vi "MenuEditor.vi"(11 "ItemsIn":T1(array[cluster])) -> (0 "Cancelled?":bool, 3 "ItemsOut":T1(array[cluster]))   [LabVIEW 2020, in "XMenuBar.xctl"]
doc: "Menu Item Editor"
uses:
  XMenuBar.xctl
panel:
  in  "Down":bool
  in  "Up":bool
  in  "Png":bool
  in  "LvSymb":i32(listbox)
  in  "PngSymb":path
  in  "IndentIn":bool
  in  "IndentOut":bool
  in  "Remove":bool
  in  "Add":bool
  in  "ItemTag":string caption="Item Tag:"
  in  "Checked":bool
  in  "ParentTag":string caption="Parent Tag(Use empty for top level menue):"
  in  "Load":bool
  in  "Name":string caption="ItemName"
  in  "Save":bool
  in  "Data":string(tree) caption="XMenu Data:"
  in  "Cancel":bool
  in  "OK":bool
  # "Item Operation"
  # "Menu File"
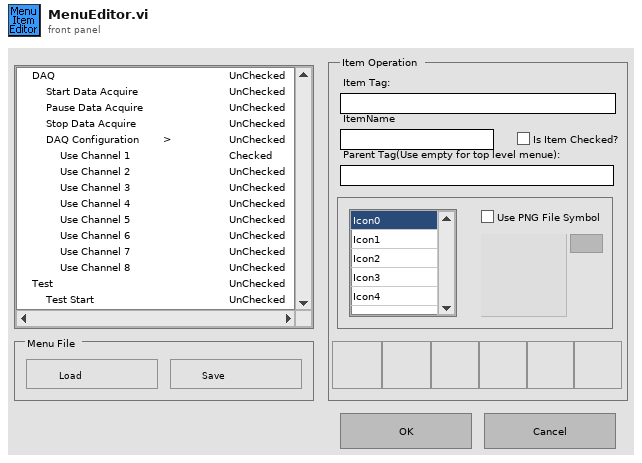
[diagram p1: front panel]
types:
  T1 = cluster{"Tag":string, "Name":string, "Index":i32, "Checked":bool, "Parent":string}[]
  T2 = enum16{"open", "replace", "create", "open or create", "replace or create", "replace or create with confirmation"}
  T3 = cluster{"Tag":string, "Name":string, "Symbol":i32, "Checked":bool, "ParentTag":string}
  T4 = enum8{"Enabled", "Disabled", "Disabled and Grayed Out"}
  T5 = typedef "imagedata.ctl" = cluster{"image type":i32, "image depth":i32, "image":u8[], "mask":u8[], "colors":u32[], "Rectangle":cluster{"left":i16, "top":i16, "right":i16, "bottom":i16}}
  T6 = cluster{string, "Cell String":string, "Glyph":i32, bool, "Navigate Tree:Get Parent":string}
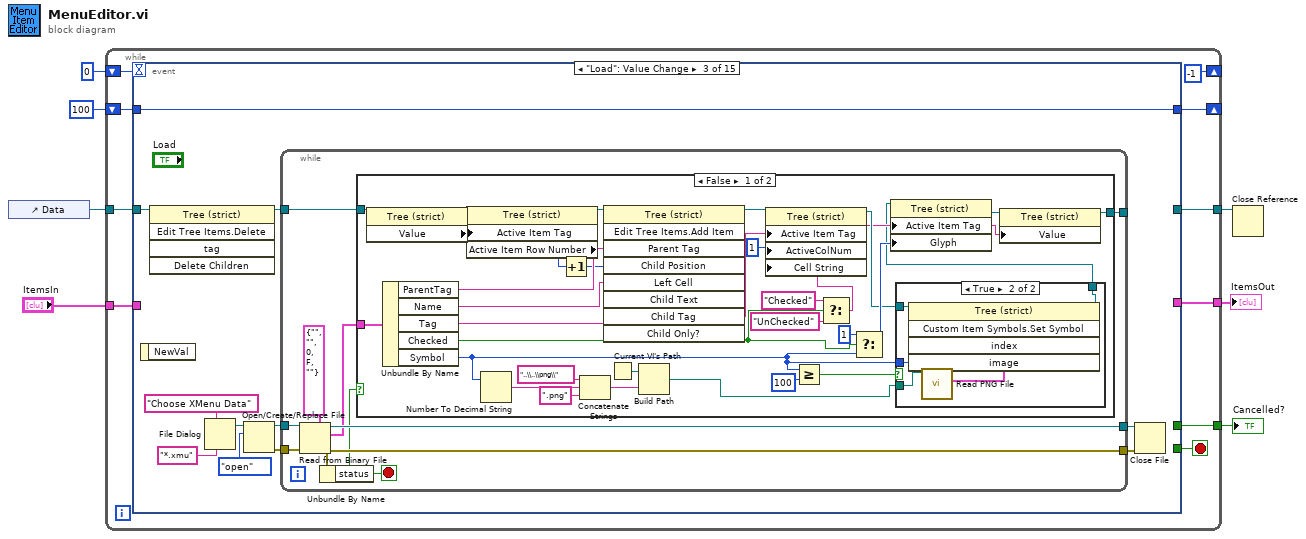
[diagram p0: block diagram]
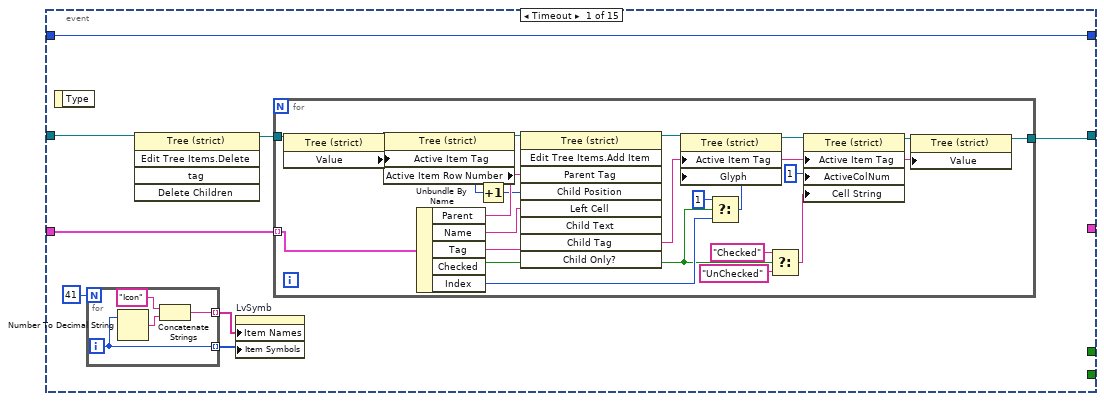
[diagram p2: hidden frame]
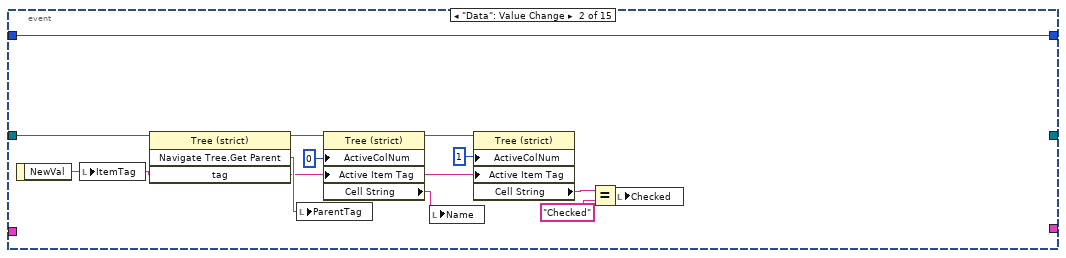
[diagram p3: hidden frame]
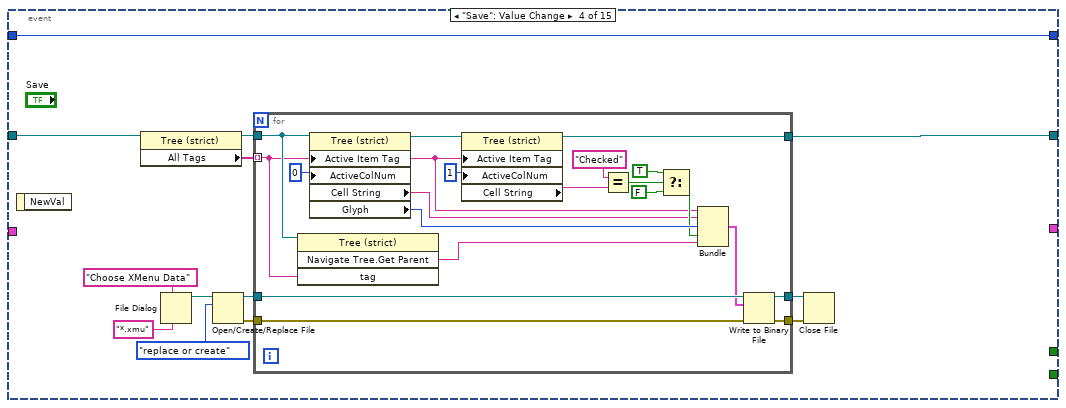
[diagram p6: hidden frame]
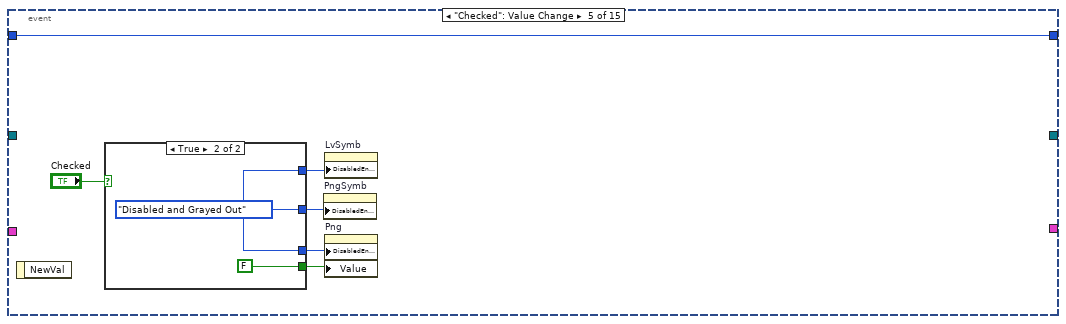
[diagram p7: hidden frame]
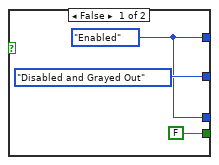
[diagram p8: hidden frame]
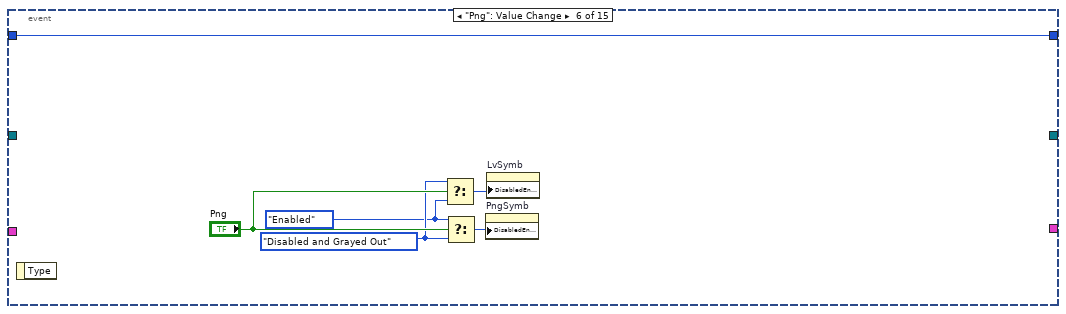
[diagram p9: hidden frame]
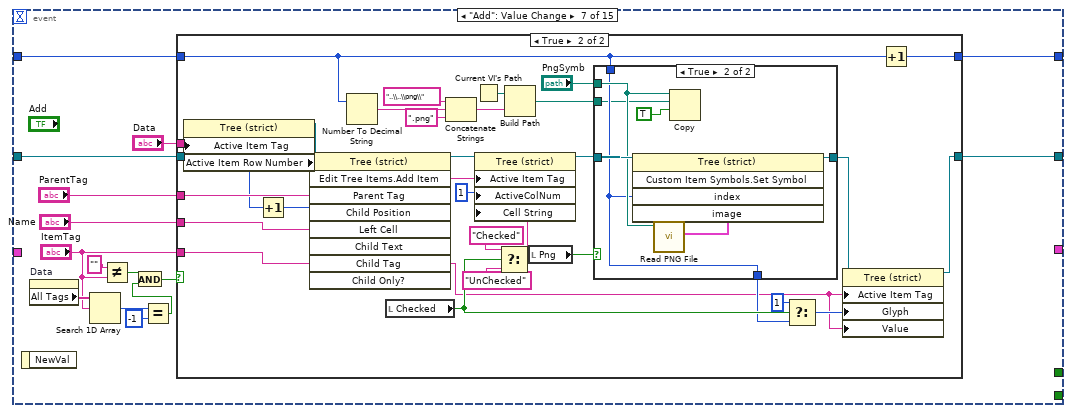
[diagram p10: hidden frame]
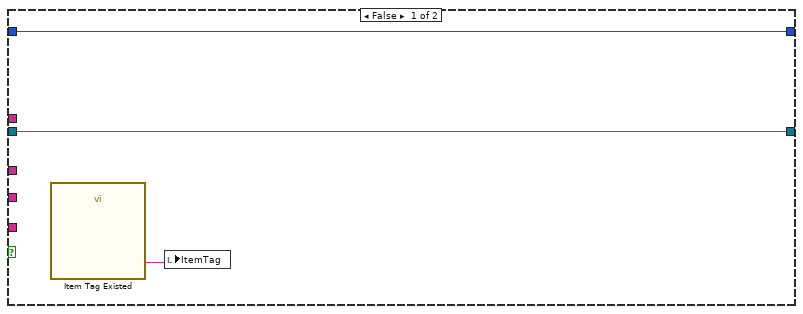
[diagram p11: hidden frame]
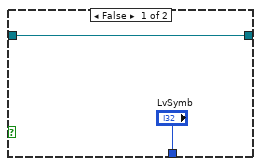
[diagram p12: hidden frame]
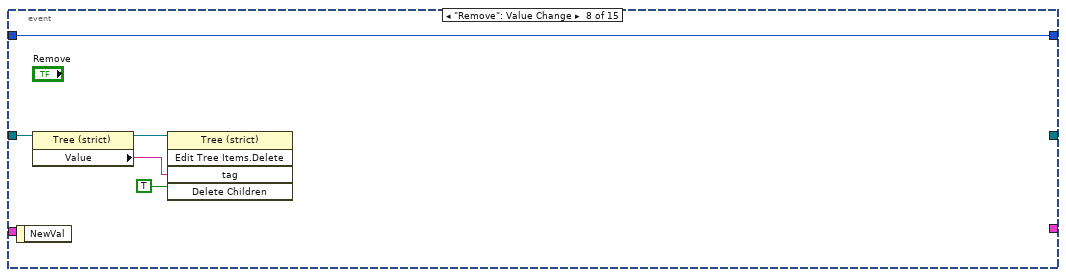
[diagram p13: hidden frame]
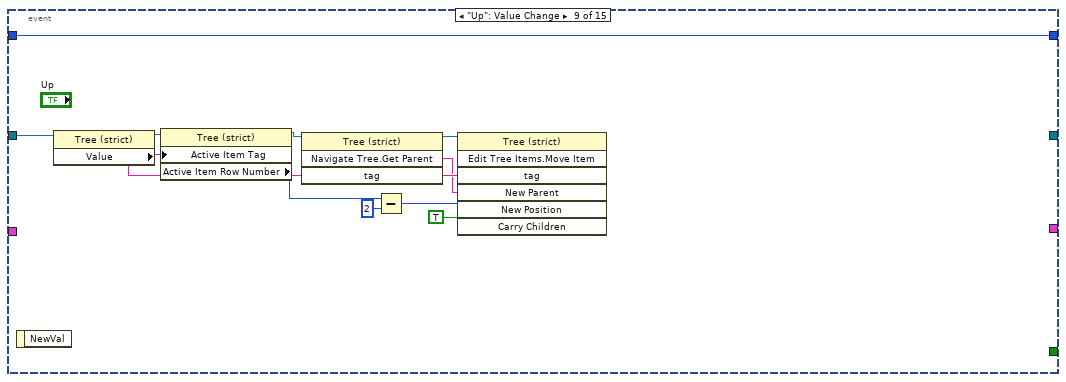
[diagram p14: hidden frame]
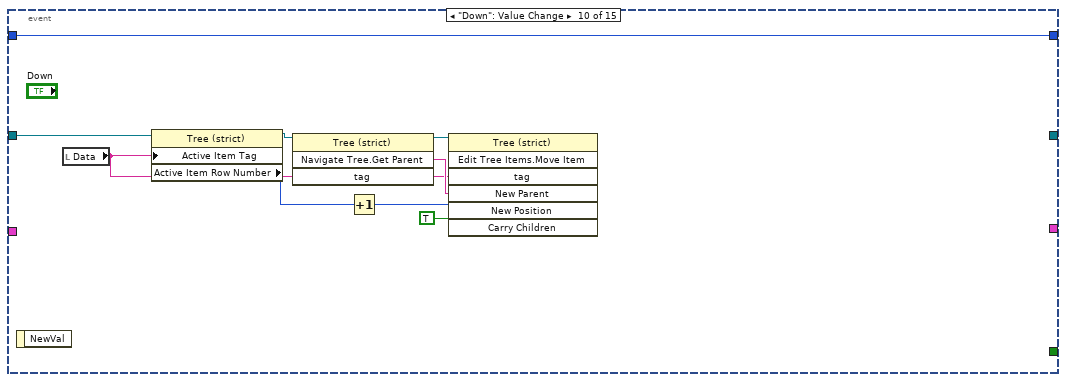
[diagram p15: hidden frame]
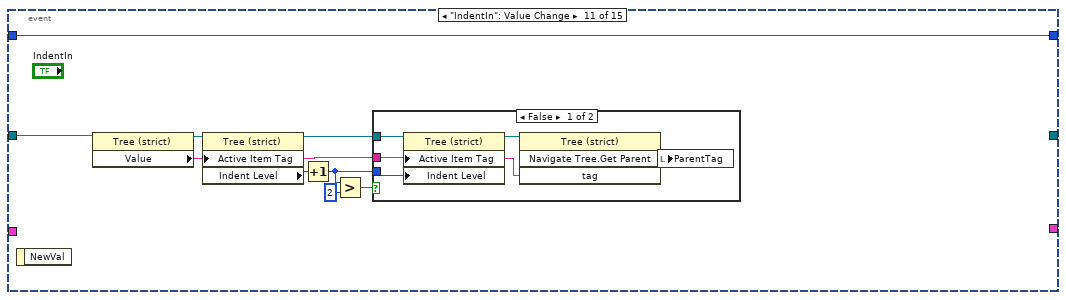
[diagram p16: hidden frame]
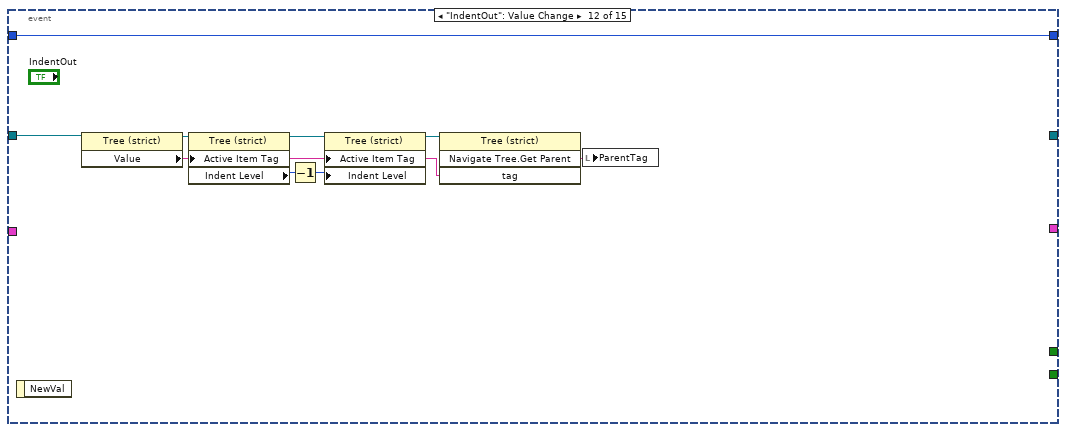
[diagram p18: hidden frame]
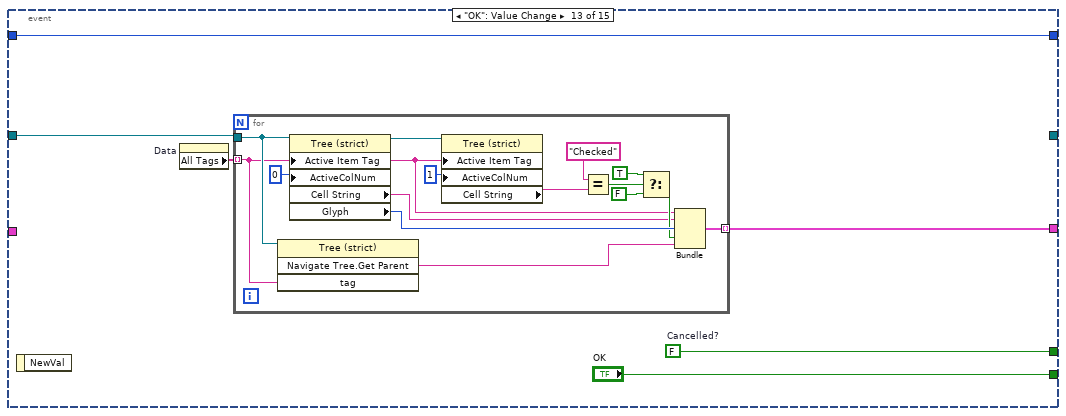
[diagram p19: hidden frame]
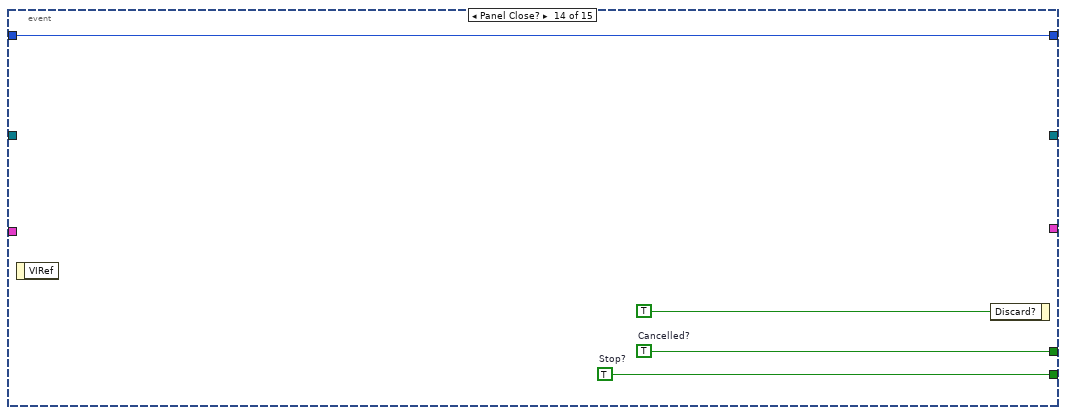
[diagram p20: hidden frame]
diagram:
  n1 = control-ref of="Data"() -> (w5:refnum<vi>)
  n2 = while {
    tunnel: [w16] -> w7
    shift-right: [-1] -> _
    shift-left: 0 -> [w14]
    tunnel: w5 -> [w13]
    shift-right: [w11] -> _
    shift-left: 100 -> [w12]
    tunnel: [w10] -> w3
    tunnel: [w9] -> w1
    tunnel: "ItemsIn" -> [w8]
    stop <- w17 stop-if-true
    n3 = event shown="[2] \"Load\": Value Change" {
      selector: _ -> [_ _ _ _ _ _ _ _ _ _ _ _ _ _ _]
      dyn-events: _ -> [_ _ _ _ _ _ _ _ _ _ _ _ _ _ _]
      timeout: w14 -> [_ _ _ _ _ _ _ _ _ _ _ _ _ _ _]
      tunnel: [_ _ _ _ _ _ _ _ _ _ _ _ "OK" w301 "Cancel"] -> w17
      tunnel: [_ _ _ _ _ _ _ _ _ _ _ _ w283 w300 w305] -> w16
      tunnel: w13 -> [w25 w63 w73 w123 _ _ w186 w234 w238 w247 w260 w277 w279 _ _]
      tunnel: w12 -> [w21 w61 w74 w134 w160 w166 w180 w232 w245 w254 w255 w272 w281 w299 w303]
      tunnel: [w21 w61 w74 w134 w160 w166 w179 w232 w245 w254 w255 w272 w281 w299 w303] -> w11
      tunnel: [w18 _ _ w122 _ _ w172 _ _ _ _ _ _ _ _] -> w10
      tunnel: [_ _ _ _ _ _ _ _ _ _ _ _ w278 _ _] -> w9
      tunnel: w8 -> [w19 _ _ _ _ _ _ _ _ _ _ _ _ _ _]
      event Timeout {
        n4 = event-data() -> ()  [unwired: 1 in, 1 out]
        n5 = for {
          N: 41 -> [_]
          tunnel: [w51] -> w22 mode=indexing
          tunnel: [w48] -> w23 mode=indexing
          i -> [w51]
          n6 = Number To Decimal String(number=w51) -> (decimal integer string=w50:string)  [unwired: 1 in]
          n7 = Concatenate Strings("Icon" ("string (\"\")"), w50) -> (w48:string)
        }
        n8 = invoke class="Tree (strict)" method="Edit Tree Items.Delete"(reference=w25) -> (reference out=w20:refnum<vi>)  [unwired: 4 in, 4 out]
        n9 = property on="LvSymb" class="LstBox (strict)"("Item Names"=w23, "Item Symbols"=w22) -> ()  [unwired: 2 in, 2 out]
        n10 = for {
          tunnel: w20 -> [w28]
          tunnel: w19 -> [w27] mode=indexing
          tunnel: [w26] -> w18
          n11 = property class="Tree (strict)"(reference=w28) -> (reference out=w30:refnum<vi>, "Value"=w29:string)  [unwired: 1 in, 1 out]
          n12 = property class="Tree (strict)"(reference=w30, "Active Item Tag"=w29) -> (reference out=w35:refnum<vi>, "Active Item Row Number"=w34:i32)  [unwired: 1 in, 1 out]
          n13 = Unbundle By Name(w27) -> ("Parent"=w47:string, "Name"=w46:string, "Tag"=w31:string, "Checked"=w37:bool, "Index"=w44:i32)
          n14 = Increment(x=w34) -> (x+1=w33:i32)
          n15 = invoke class="Tree (strict)" method="Edit Tree Items.Add Item"(reference=w35, "Parent Tag"=w47, "Child Position"=w33, "Left Cell"=w46, "Child Tag"=w31) -> (reference out=w45:refnum<vi>)  [unwired: 4 in, 8 out]
          n16 = Select(t=1, s=w37, f=w44) -> (s? t:f=w42:i32)
          n17 = property class="Tree (strict)"(reference=w45, "Active Item Tag"=w31, "Glyph"=w42) -> (reference out=w38:refnum<vi>)  [unwired: 1 in, 1 out]
          n18 = Select(t="Checked" ("Active Cell:String"), s=w37, f="UnChecked") -> (s? t:f=w36:string)
          n19 = property class="Tree (strict)"(reference=w38, "Active Item Tag"=w31, "ActiveColNum"=1 ("Active Cell:Active Column Number"), "Cell String"=w36) -> (reference out=w32:refnum<vi>)  [unwired: 1 in, 1 out]
          n20 = property class="Tree (strict)"(reference=w32, "Value"=w31) -> (reference out=w26:refnum<vi>)  [unwired: 1 in, 1 out]
        }
      }
      event "Data": Value Change {
        n21 = event-data() -> ("NewVal"=w55:string)  [unwired: 1 in]
        n22 = local write "ItemTag"(w55) -> ()
        n23 = invoke class="Tree (strict)" method="Navigate Tree.Get Parent"(reference=w63, "tag"=w55) -> (reference out=w60:refnum<vi>, "Navigate Tree:Get Parent"=w62:string)  [unwired: 2 in, 2 out]
        n24 = local write "ParentTag"(w62) -> ()
        n25 = property class="Tree (strict)"(reference=w60, "ActiveColNum"=0 ("Active Cell:Active Column Number"), "Active Item Tag"=w55) -> (reference out=w57:refnum<vi>, "Cell String"=w58:string)  [unwired: 1 in, 1 out]
        n26 = local write "Name"(w58) -> ()
        n27 = property class="Tree (strict)"(reference=w57, "ActiveColNum"=1 ("Active Cell:Active Column Number"), "Active Item Tag"=w55) -> ("Cell String"=w54:string)  [unwired: 1 in, 2 out]
        n28 = Equal?(x=w54, y="Checked") -> (x = y?=w52:bool)
        n29 = local write "Checked"(w52) -> ()
      }
      event "Load": Value Change {
        n30 = event-data() -> ()  [unwired: 1 in, 1 out]
        n31 = invoke class="Tree (strict)" method="Edit Tree Items.Delete"(reference=w73) -> (reference out=w70:refnum<vi>)  [unwired: 4 in, 4 out]
        n32 = File Dialog(6:"*.xmu" ("pattern (all files)"), 7:"Choose XMenu Data" ("Prompt")) -> (3:w65:path)  [unwired: 5 in, 3 out]
        n33 = Open/Create/Replace File(file path (use dialog)=w65, operation (0:open)=T2."open") -> (refnum out=w67:refnum<file>, error out=w66:errorcluster)  [unwired: 4 in, 1 out]
        n34 = while {
          tunnel: [w81] -> w69
          tunnel: w67 -> [w83]
          tunnel: w66 -> [w82]
          tunnel: [w78] -> w68
          tunnel: w70 -> [w75]
          tunnel: [w76] -> _
          stop <- w77 stop-if-true
          n35 = Read from Binary File(5:T3 {"Tag"="", "Name"="", "Symbol"=0, "Checked"=FALSE, "ParentTag"=""} ("Item"), 8:w82, 11:w83) -> (0:w78:errorcluster, 2:w79:T3, 3:w81:refnum<file>)  [unwired: 3 in, 1 out]
          n36 = Unbundle By Name(w78) -> ("status"=w77:bool)
          n37 = case shown="False" w77 {
            tunnel: w79 -> [w114 _]
            tunnel: [w105 w121] -> w76
            tunnel: w75 -> [w104 w121]
            frame False {
              n38 = property class="Tree (strict)"(reference=w104) -> (reference out=w103:refnum<vi>, "Value"=w102:string)  [unwired: 1 in, 1 out]
              n39 = Unbundle By Name(w114) -> ("ParentTag"=w113:string, "Name"=w112:string, "Tag"=w87:string, "Checked"=w88:bool, "Symbol"=w85:i32)
              n40 = property class="Tree (strict)"(reference=w103, "Active Item Tag"=w102) -> (reference out=w108:refnum<vi>, "Active Item Row Number"=w107:i32)  [unwired: 1 in, 1 out]
              n41 = Number To Decimal String(number=w85) -> (decimal integer string=w101:string)  [unwired: 1 in]
              n42 = Increment(x=w107) -> (x+1=w106:i32)
              n43 = Concatenate Strings("..\\..\\png\\" ("name or relative path"), w101, ".png" ("string")) -> (w97:string)
              n44 = invoke class="Tree (strict)" method="Edit Tree Items.Add Item"(reference=w108, "Parent Tag"=w113, "Child Position"=w106, "Left Cell"=w112, "Child Tag"=w87) -> (reference out=w91:refnum<vi>)  [unwired: 4 in, 8 out]
              n45 = Current VI's Path() -> (path=w98:path)
              n46 = Build Path(base path=w98, name or relative path=w97) -> (appended path=w84:path)
              n47 = Greater Or Equal?(x=w85, y=100) -> (x >= y?=w94:bool)
              n48 = Select(t="Checked" ("Active Cell:String"), s=w88, f="UnChecked") -> (s? t:f=w109:string)
              n49 = property class="Tree (strict)"(reference=w91, "Active Item Tag"=w87, "ActiveColNum"=1 ("Active Cell:Active Column Number"), "Cell String"=w109) -> (reference out=w89:refnum<vi>)  [unwired: 1 in, 1 out]
              n50 = Select(t=1, s=w88, f=w85) -> (s? t:f=w92:i32)
              n51 = case shown="True" w94 {
                tunnel: w89 -> [w115 w119]
                tunnel: w85 -> [_ w118]
                tunnel: [w115 w117] -> w86
                tunnel: w84 -> [_ w116]
                frame False {
                }
                frame True {
                  n52 = call <vilib>:"Read PNG File.vi"("path to PNG file"=w116) -> ("image data"=w120:T5)  [unwired: 8 in, 2 out]
                  n53 = invoke class="Tree (strict)" method="Custom Item Symbols.Set Symbol"(reference=w119, "index"=w118, "image"=w120) -> (reference out=w117:refnum<vi>)  [unwired: 2 in, 4 out]
                }
              }
              n54 = property class="Tree (strict)"(reference=w86, "Active Item Tag"=w87, "Glyph"=w92) -> (reference out=w90:refnum<vi>)  [unwired: 1 in, 1 out]
              n55 = property class="Tree (strict)"(reference=w90, "Value"=w87) -> (reference out=w105:refnum<vi>)  [unwired: 1 in, 1 out]
            }
            frame True {
            }
          }
        }
        n56 = Close File(refnum=w69, error in=w68) -> ()  [unwired: 2 out]
      }
      event "Save": Value Change {
        n57 = event-data() -> ()  [unwired: 1 in, 1 out]
        n58 = property class="Tree (strict)"(reference=w123) -> (reference out=w132:refnum<vi>, "All Tags"=w133:string[])  [unwired: 1 in, 1 out]
        n59 = File Dialog(6:"*.xmu" ("pattern (all files)"), 7:"Choose XMenu Data" ("Prompt")) -> (3:w126:path)  [unwired: 5 in, 3 out]
        n60 = Open/Create/Replace File(file path (use dialog)=w126, operation (0:open)=T2."replace or create") -> (refnum out=w129:refnum<file>, error out=w128:errorcluster)  [unwired: 4 in, 1 out]
        n61 = for {
          tunnel: w133 -> [w139] mode=indexing
          tunnel: w128 -> [w153]
          tunnel: w129 -> [w154]
          tunnel: w132 -> [w150]
          tunnel: [w141] -> w130
          tunnel: [w140] -> w131
          tunnel: [w135] -> w122
          n62 = invoke class="Tree (strict)" method="Navigate Tree.Get Parent"(reference=w150, "tag"=w139) -> ("Navigate Tree:Get Parent"=w136:string)  [unwired: 2 in, 3 out]
          n63 = property class="Tree (strict)"(reference=w150, "Active Item Tag"=w139, "ActiveColNum"=0 ("Active Cell:Active Column Number")) -> (reference out=w152:refnum<vi>, "Cell String"=w138:string, "Glyph"=w144:i32)  [unwired: 1 in, 1 out]
          n64 = property class="Tree (strict)"(reference=w152, "Active Item Tag"=w139, "ActiveColNum"=1 ("Active Cell:Active Column Number")) -> (reference out=w135:refnum<vi>, "Cell String"=w145:string)  [unwired: 1 in, 1 out]
          n65 = Equal?(x="Checked" ("y"), y=w145) -> (x = y?=w149:bool)
          n66 = Select(t=TRUE, s=w149, f=FALSE) -> (s? t:f=w143:bool)
          n67 = Bundle(w139, "Cell String"=w138, "Glyph"=w144, w143, "Navigate Tree:Get Parent"=w136) -> (w142:T6)  [unwired: 1 in]
          n68 = Write to Binary File(file (use dialog)=w154, data=w142, error in=w153) -> (refnum out=w141:refnum<file>, error out=w140:errorcluster)  [unwired: 3 in, 1 out]
        }
        n69 = Close File(refnum=w130, error in=w131) -> ()  [unwired: 2 out]
      }
      event "Checked": Value Change {
        n70 = event-data() -> ()  [unwired: 1 in, 1 out]
        n71 = case shown="True" "Checked" {
          tunnel: [w162 w165] -> w158
          tunnel: [T4."Disabled and Grayed Out" ("Disabled") w165] -> w157
          tunnel: [w162 w165] -> w156
          tunnel: [FALSE ("Png") FALSE ("Png")] -> w155
          frame False {
            w162 = T4."Enabled" ("Disabled")
          }
          frame True {
            w165 = T4."Disabled and Grayed Out" ("Disabled")
          }
        }
        n72 = property on="PngSymb" class="Path"("DisabledEnum"=w157) -> ()  [unwired: 2 in, 2 out]
        n73 = property on="LvSymb" class="LstBox (strict)"("DisabledEnum"=w158) -> ()  [unwired: 2 in, 2 out]
        n74 = property on="Png" class="Bool (strict)"("DisabledEnum"=w156, "Value"=w155) -> ()  [unwired: 2 in, 2 out]
      }
      event "Png": Value Change {
        w168 = T4."Disabled and Grayed Out" ("Disabled")
        w167 = T4."Enabled" ("Disabled")
        n75 = event-data() -> ()  [unwired: 1 in, 1 out]
        n76 = Select(t=w168, s="Png", f=w167) -> (s? t:f=w169:T4)
        n77 = Select(t=w167, s="Png", f=w168) -> (s? t:f=w171:T4)
        n78 = property on="PngSymb" class="Path"("DisabledEnum"=w171) -> ()  [unwired: 2 in, 2 out]
        n79 = property on="LvSymb" class="LstBox (strict)"("DisabledEnum"=w169) -> ()  [unwired: 2 in, 2 out]
      }
      event "Add": Value Change {
        n80 = event-data() -> ()  [unwired: 1 in, 1 out]
        n81 = property on="Data" class="Tree (strict)"() -> ("All Tags"=w183:string[])  [unwired: 2 in, 2 out]
        n82 = Search 1D Array(1D array=w183, element="ItemTag") -> (index of element=w182:i32)  [unwired: 1 in]
        n83 = Not Equal?(x="", y="ItemTag") -> (x != y?=w176:bool)
        n84 = Equal?(x=w182, y=-1) -> (x = y?=w175:bool)
        n85 = And(x=w176, y=w175) -> (x .and. y?=w174:bool)
        n86 = case shown="True" w174 {
          tunnel: w186 -> [w187 w202]
          tunnel: "ParentTag" -> [_ w220]
          tunnel: "Name" -> [_ w215]
          tunnel: "ItemTag" -> [_ w199]
          tunnel: [w188 w219] -> w179
          tunnel: w180 -> [w188 w191]
          tunnel: "Data" -> [_ w204]
          tunnel: [w187 w198] -> w172
          frame False {
            n87 = call "Item Tag Existed"() -> ("Item Tag:"=w189:string)  [unwired: 17 in, 2 out]
            n88 = local write "ItemTag"(w189) -> ()
          }
          frame True {
            n89 = property class="Tree (strict)"(reference=w202, "Active Item Tag"=w204) -> (reference out=w203:refnum<vi>, "Active Item Row Number"=w201:i32)  [unwired: 1 in, 1 out]
            n90 = Increment(x=w201) -> (x+1=w200:i32)
            n91 = invoke class="Tree (strict)" method="Edit Tree Items.Add Item"(reference=w203, "Parent Tag"=w220, "Child Position"=w200, "Left Cell"=w215, "Child Tag"=w199) -> (reference out=w205:refnum<vi>, "Edit Tree Items:Add Item"=w206:string)  [unwired: 4 in, 7 out]
            n92 = Number To Decimal String(number=w191) -> (decimal integer string=w196:string)  [unwired: 1 in]
            n93 = local read "Checked"() -> (w208:bool)
            n94 = Concatenate Strings("..\\..\\png\\" ("name or relative path"), w196, ".png" ("string")) -> (w192:string)
            n95 = Current VI's Path() -> (path=w193:path)
            n96 = Select(t="Checked" ("Active Cell:String"), s=w208, f="UnChecked") -> (s? t:f=w216:string)
            n97 = property class="Tree (strict)"(reference=w205, "Active Item Tag"=w206, "ActiveColNum"=1 ("Active Cell:Active Column Number"), "Cell String"=w216) -> (reference out=w212:refnum<vi>)  [unwired: 1 in, 1 out]
            n98 = Build Path(base path=w193, name or relative path=w192) -> (appended path=w190:path)
            n99 = local read "Png"() -> (w213:bool)
            n100 = case shown="True" w213 {
              tunnel: w212 -> [w222 w228]
              tunnel: w191 -> [_ w224]
              tunnel: [w222 w227] -> w209
              tunnel: ["LvSymb" w224] -> w207
              tunnel: "PngSymb" -> [_ w226]
              tunnel: w190 -> [_ w223]
              frame False {
              }
              frame True {
                n101 = call <vilib>:"Read PNG File.vi"("path to PNG file"=w226) -> ("image data"=w229:T5)  [unwired: 8 in, 2 out]
                n102 = invoke class="Tree (strict)" method="Custom Item Symbols.Set Symbol"(reference=w228, "index"=w224, "image"=w229) -> (reference out=w227:refnum<vi>)  [unwired: 2 in, 4 out]
                n103 = Copy(9:TRUE ("overwrite (F)"), 10:w223, 11:w226) -> ()  [unwired: 2 in, 3 out]
              }
            }
            n104 = Select(t=1, s=w208, f=w207) -> (s? t:f=w210:i32)
            n105 = property class="Tree (strict)"(reference=w209, "Active Item Tag"=w199, "Glyph"=w210, "Value"=w199) -> (reference out=w198:refnum<vi>)  [unwired: 1 in, 1 out]
            n106 = Increment(x=w191) -> (x+1=w219:i32)
          }
        }
      }
      event "Remove": Value Change {
        n107 = event-data() -> ()  [unwired: 1 in, 1 out]
        n108 = property class="Tree (strict)"(reference=w234) -> (reference out=w231:refnum<vi>, "Value"=w230:string)  [unwired: 1 in, 1 out]
        n109 = invoke class="Tree (strict)" method="Edit Tree Items.Delete"(reference=w231, "tag"=w230, "Delete Children"=TRUE ("Delete Children?")) -> ()  [unwired: 2 in, 5 out]
      }
      event "Up": Value Change {
        n110 = event-data() -> ()  [unwired: 1 in, 1 out]
        n111 = property class="Tree (strict)"(reference=w238) -> (reference out=w237:refnum<vi>, "Value"=w236:string)  [unwired: 1 in, 1 out]
        n112 = property class="Tree (strict)"(reference=w237, "Active Item Tag"=w236) -> (reference out=w239:refnum<vi>, "Active Item Row Number"=w241:i32)  [unwired: 1 in, 1 out]
        n113 = invoke class="Tree (strict)" method="Navigate Tree.Get Parent"(reference=w239, "tag"=w236) -> (reference out=w240:refnum<vi>, "Navigate Tree:Get Parent"=w235:string)  [unwired: 2 in, 2 out]
        n114 = Subtract(x=w241, y=2) -> (x-y=w243:i32)
        n115 = invoke class="Tree (strict)" method="Edit Tree Items.Move Item"(reference=w240, "tag"=w236, "New Parent"=w235, "New Position"=w243, "Carry Children"=TRUE ("Carry Children?")) -> ()  [unwired: 2 in, 7 out]
      }
      event "Down": Value Change {
        n116 = event-data() -> ()  [unwired: 1 in, 1 out]
        n117 = local read "Data"() -> (w246:string)
        n118 = property class="Tree (strict)"(reference=w247, "Active Item Tag"=w246) -> (reference out=w251:refnum<vi>, "Active Item Row Number"=w250:i32)  [unwired: 1 in, 1 out]
        n119 = invoke class="Tree (strict)" method="Navigate Tree.Get Parent"(reference=w251, "tag"=w246) -> (reference out=w252:refnum<vi>, "Navigate Tree:Get Parent"=w248:string)  [unwired: 2 in, 2 out]
        n120 = Increment(x=w250) -> (x+1=w249:i32)
        n121 = invoke class="Tree (strict)" method="Edit Tree Items.Move Item"(reference=w252, "tag"=w246, "New Parent"=w248, "New Position"=w249, "Carry Children"=TRUE ("Carry Children?")) -> ()  [unwired: 2 in, 7 out]
      }
      event "IndentIn": Value Change {
        n122 = event-data() -> ()  [unwired: 1 in, 1 out]
        n123 = property class="Tree (strict)"(reference=w260) -> (reference out=w263:refnum<vi>, "Value"=w262:string)  [unwired: 1 in, 1 out]
        n124 = property class="Tree (strict)"(reference=w263, "Active Item Tag"=w262) -> (reference out=w261:refnum<vi>, "Indent Level"=w257:i32)  [unwired: 1 in, 1 out]
        n125 = Increment(x=w257) -> (x+1=w256:i32)
        n126 = Greater?(x=w256, y=2) -> (0:w258:bool)
        n127 = case shown="False" w258 {
          tunnel: w262 -> [w265 _]
          tunnel: w261 -> [w268 _]
          tunnel: w256 -> [w267 _]
          frame False {
            n128 = property class="Tree (strict)"(reference=w268, "Active Item Tag"=w265, "Indent Level"=w267) -> (reference out=w266:refnum<vi>)  [unwired: 1 in, 1 out]
            n129 = invoke class="Tree (strict)" method="Navigate Tree.Get Parent"(reference=w266, "tag"=w265) -> ("Navigate Tree:Get Parent"=w264:string)  [unwired: 2 in, 3 out]
            n130 = local write "ParentTag"(w264) -> ()
          }
          frame True {
          }
        }
      }
      event "IndentOut": Value Change {
        n131 = event-data() -> ()  [unwired: 1 in, 1 out]
        n132 = property class="Tree (strict)"(reference=w277) -> (reference out=w275:refnum<vi>, "Value"=w270:string)  [unwired: 1 in, 1 out]
        n133 = property class="Tree (strict)"(reference=w275, "Active Item Tag"=w270) -> (reference out=w274:refnum<vi>, "Indent Level"=w276:i32)  [unwired: 1 in, 1 out]
        n134 = Decrement(x=w276) -> (x-1=w273:i32)
        n135 = property class="Tree (strict)"(reference=w274, "Active Item Tag"=w270, "Indent Level"=w273) -> (reference out=w271:refnum<vi>)  [unwired: 1 in, 1 out]
        n136 = invoke class="Tree (strict)" method="Navigate Tree.Get Parent"(reference=w271, "tag"=w270) -> ("Navigate Tree:Get Parent"=w269:string)  [unwired: 2 in, 3 out]
        n137 = local write "ParentTag"(w269) -> ()
      }
      event "OK": Value Change {
        w283 = FALSE  # Cancelled?
        n138 = event-data() -> ()  [unwired: 1 in, 1 out]
        n139 = property on="Data" class="Tree (strict)"() -> ("All Tags"=w280:string[])  [unwired: 2 in, 2 out]
        n140 = for {
          tunnel: w280 -> [w288] mode=indexing
          tunnel: w279 -> [w296]
          tunnel: [w285] -> w278 mode=indexing
          n141 = invoke class="Tree (strict)" method="Navigate Tree.Get Parent"(reference=w296, "tag"=w288) -> ("Navigate Tree:Get Parent"=w284:string)  [unwired: 2 in, 3 out]
          n142 = property class="Tree (strict)"(reference=w296, "Active Item Tag"=w288, "ActiveColNum"=0 ("Active Cell:Active Column Number")) -> (reference out=w298:refnum<vi>, "Cell String"=w287:string, "Glyph"=w290:i32)  [unwired: 1 in, 1 out]
          n143 = property class="Tree (strict)"(reference=w298, "Active Item Tag"=w288, "ActiveColNum"=1 ("Active Cell:Active Column Number")) -> ("Cell String"=w291:string)  [unwired: 1 in, 2 out]
          n144 = Equal?(x="Checked" ("y"), y=w291) -> (x = y?=w295:bool)
          n145 = Select(t=TRUE, s=w295, f=FALSE) -> (s? t:f=w289:bool)
          n146 = Bundle(w288, "Cell String"=w287, "Glyph"=w290, w289, "Navigate Tree:Get Parent"=w284) -> (w285:T6)  [unwired: 1 in]
        }
      }
      event Panel Close? {
        w300 = TRUE  # Cancelled?
        w301 = TRUE  # Stop?
        n147 = event-data() -> ()  [unwired: 1 in, 1 out]
        n148 = event-data("Discard?"=TRUE) -> ()  [unwired: 1 in, 1 out]
      }
      event "Cancel": Value Change {
        w305 = TRUE  # Cancelled?
        n149 = event-data() -> ()  [unwired: 1 in, 1 out]
      }
    }
  }
  "Cancelled?" <- w7
  "ItemsOut" <- w1
  n150 = Close Reference(reference=w3) -> ()  [unwired: 1 in, 1 out]
